vi "Test data.vi"() -> ()   [LabVIEW 2013]
panel:
  in  "Right ROI":T1={"Global Rectangle"=[735, 244, 1004, 747], "Contours"=[{"ID"=enum."External", "Type"=7, "Coordinates"=[736, 512, 169, 267, 299258, 90000]}]} {"Contours"."Type" items=["No Selection", "Point", "Line", "Rectangle", "Oval", "Polygon", "Freehand Region", "Annulus", "Unused2", "Unused3", "Broken Line", "Freehand Line", "Rotated Rectangle"]}
  in  "Left ROI":T1={"Global Rectangle"=[140, 153, 435, 722], "Contours"=[{"ID"=enum."External", "Type"=7, "Coordinates"=[471, 481, 245, 331, 98891, 226332]}]} {"Contours"."Type" items=["No Selection", "Point", "Line", "Rectangle", "Oval", "Polygon", "Freehand Region", "Annulus", "Unused2", "Unused3", "Broken Line", "Freehand Line", "Rotated Rectangle"]}
  out "error out":errorcluster
  out "Image":T2(plugin-control)
  out "Frame #":i32
  in  "Frame":i32(c297)
  in  "stop":bool
  in  "Path":path=path "C:/Users/achiu/Desktop/Downloads/test_1000Frames.avi"
  out "Right Wingbeat Avg Graph":u8[](graph)
  out "Left Wingbeat Avg Graph":u8[](graph)
  in  "[Average Sector Data]":u8[][](array[numeric])=array500x32[16000 elements]
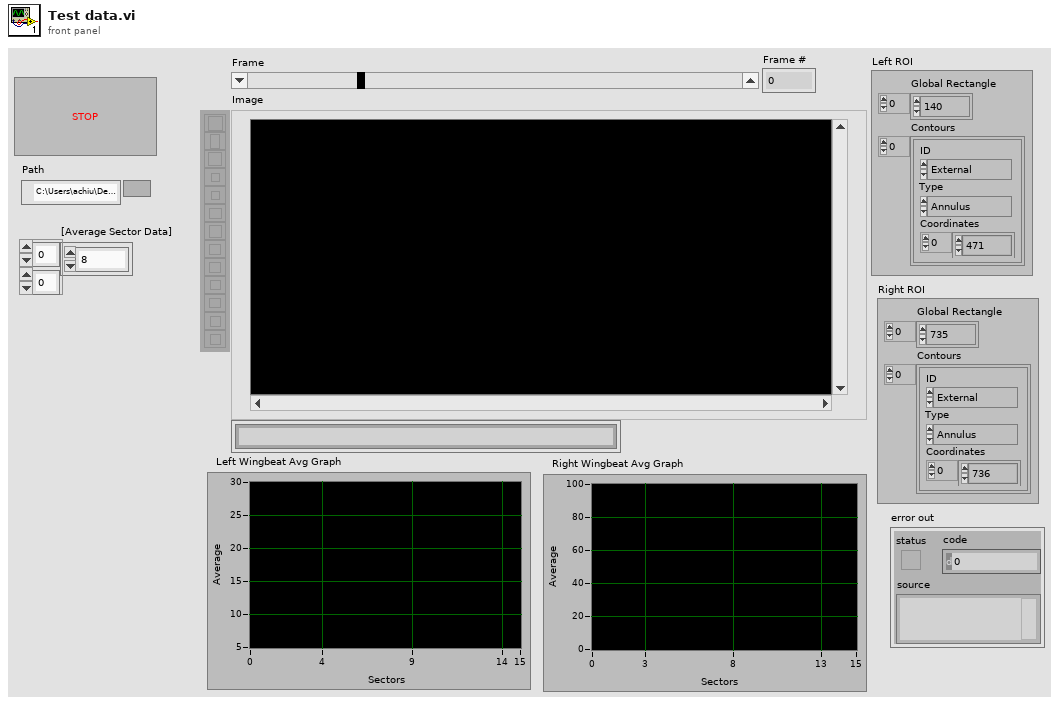
[diagram p1: front panel]
types:
  T1 = typedef "ROI Descriptor" = cluster{"Global Rectangle":i32[], "Contours":cluster{"ID":enum32{"External", "Internal"}, "Type":u32, "Coordinates":i32[]}[]}
  T2 = typedef "IMAQ Image.ctl" = refnum<image>
  T3 = typedef "Image Type" = u32
  T4 = typedef "IMAQ AVI2 Refnum.ctl" = refnum<k20>
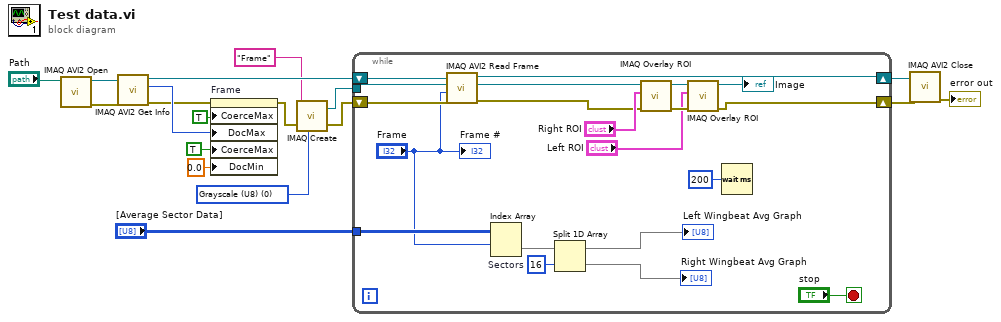
[diagram p0: block diagram]
diagram:
  w5 = T3 0 items=["Grayscale (U8)", "Grayscale (I16)", "Grayscale (SGL)", "Complex (CSG)", "RGB (U32)", "HSL (U32)", "RGB (U64)", "Grayscale (U16)"] ("Image Type")
  n1 = call "IMAQ AVI2 Open"("AVI File Path"="Path") -> ("error out"=w17:errorcluster, "AVI Refnum"=w16:T4)  [unwired: 9 in]
  n2 = call "IMAQ AVI2 Get Info"("error in (no error)"=w17, "AVI Refnum"=w16) -> ("error out"=w13:errorcluster, "Number of Frames"=w14:u32, "AVI Refnum (duplicate)"=w12:T4)  [unwired: 5 in, 2 out]
  n3 = property on="Frame" class="Scroll (strict)"(error in=w13, "CoerceMax"=TRUE ("Coerce Maximum Value"), "DocMax"=w14, "CoerceMax"=TRUE ("Coerce Maximum Value"), "DocMin"=0.0 ("Doc Min")) -> (error out=w8:errorcluster)  [unwired: 1 in, 1 out]
  n4 = call "IMAQ Create"("Image Name"="Frame", "Image Type"=w5, "error in (no error)"=w8) -> ("New Image"=w4:T2, "error out"=w7:errorcluster)  [unwired: 2 in]
  n5 = while {
    shift-right: [w19] -> w3
    shift-left: w7 -> [w32]
    tunnel: "[Average Sector Data]" -> [w37]
    tunnel: w4 -> [w29]
    shift-right: [w28] -> w2
    shift-left: w12 -> [w31]
    stop <- "stop" stop-if-true
    w35 = 16  # Sectors
    n6 = call "IMAQ AVI2 Read Frame"("error in (no error)"=w32, "Frame Number"="Frame", "Image"=w29, "AVI Refnum"=w31) -> ("error out"=w20:errorcluster, "Image Out"=w26:T2, "AVI Refnum (duplicate)"=w28:T4)  [unwired: 5 in]
    n7 = Index Array(array=w37, index (row)="Frame") -> (element=w36:u8[])  [unwired: 1 in]
    n8 = Split 1D Array(array=w36, index=w35) -> (first subarray=→"Left Wingbeat Avg Graph":u8[], second subarray=→"Right Wingbeat Avg Graph":u8[])
    n9 = call "IMAQ Overlay ROI"("error in (no error)"=w20, "ROI Descriptor"="Right ROI", "Image"=w26) -> ("error out"=w24:errorcluster, "Image Out"=w23:T2)  [unwired: 7 in]
    n10 = call "IMAQ Overlay ROI"("error in (no error)"=w24, "ROI Descriptor"="Left ROI", "Image"=w23) -> ("error out"=w19:errorcluster, "Image Out"=→"Image":T2)  [unwired: 7 in]
    n11 = Wait (ms)(milliseconds to wait=u32 200) -> ()  [unwired: 1 out]
    "Frame #" <- "Frame"
  }
  n12 = call "IMAQ AVI2 Close"("error in (no error)"=w3, "AVI Refnum"=w2) -> ("error out"=→"error out":errorcluster)  [unwired: 9 in]
